vi "U8 array to U32 array.vi"(11 "Array in":u8[](array[numeric])) -> (3 "Array out":u32[](array[numeric]))   [LabVIEW 2020, in "wamplv.lvlib" / "Utils.lvclass"]
uses:
  Utils.lvclass
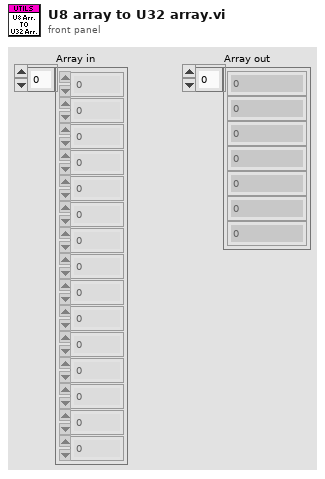
[diagram p1: front panel]
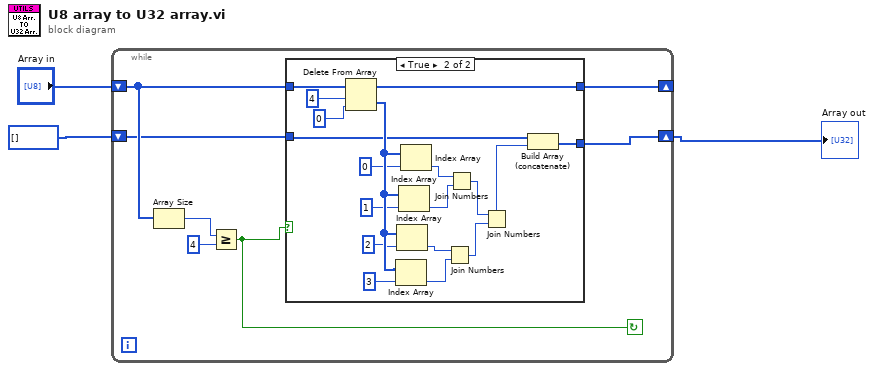
[diagram p0: block diagram]
diagram:
  n1 = while {
    shift-right: [w10] -> _
    shift-left: "Array in" -> [w9]
    shift-right: [w4] -> w1
    shift-left: u32[] [] -> [w5]
    stop <- w6 continue-if-true
    n2 = Array Size(array=w9) -> (size(s)=w8:i32)
    n3 = Greater Or Equal?(x=w8, y=4) -> (x >= y?=w6:bool)
    n4 = case shown="True" w6 {
      tunnel: w9 -> [w12 w30]
      tunnel: [w12 w16] -> w10
      tunnel: w5 -> [w11 w15]
      tunnel: [w11 w14] -> w4
      frame False {
      }
      frame True {
        n5 = Delete From Array(array=w30, length=4, index=0) -> (deleted portion=w27:u8[], array with subset deleted=w16:u8[])
        n6 = Index Array(array=w27, index=3) -> (element=w19:u8)
        n7 = Index Array(array=w27, index=2) -> (element=w20:u8)
        n8 = Index Array(array=w27, index=1) -> (element=w21:u8)
        n9 = Index Array(array=w27, index=0) -> (element=w22:u8)
        n10 = Join Numbers(hi=w20, lo=w19) -> ((hi.lo)=w17:u16)
        n11 = Join Numbers(hi=w22, lo=w21) -> ((hi.lo)=w18:u16)
        n12 = Join Numbers(hi=w18, lo=w17) -> ((hi.lo)=w13:u32)
        n13 = Build Array (concatenate)(w15, w13) -> (w14:u32[])
      }
    }
  }
  "Array out" <- w1
